vi "DSPS_E36000.Get ID.vi"(8 "error in":errorcluster, 11 "VISA Alias":refnum<visa-resource-name>) -> (0 "error out":errorcluster, 1 "SN":string, 2 "Model":string, 3 "VISA Alias Dup":refnum<visa-resource-name>, 4 "FW":string, 5 "Mfg":string)   [LabVIEW 2018]
panel:
  out "IDN Data":string
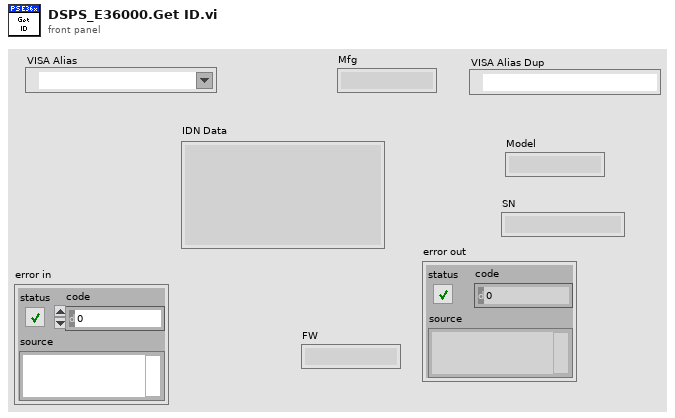
[diagram p1: front panel]
types:
  T1 = cluster{"Mfg":string, "Model":string, "SN":string, "FW":string}
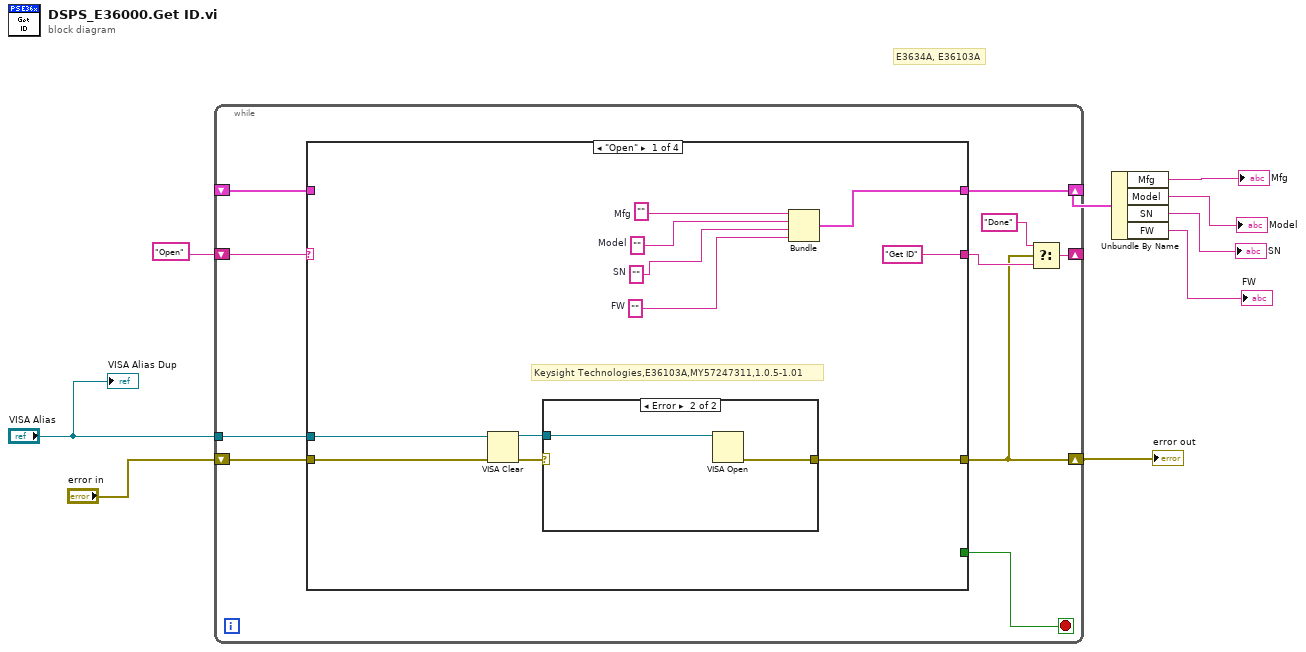
[diagram p0: block diagram]
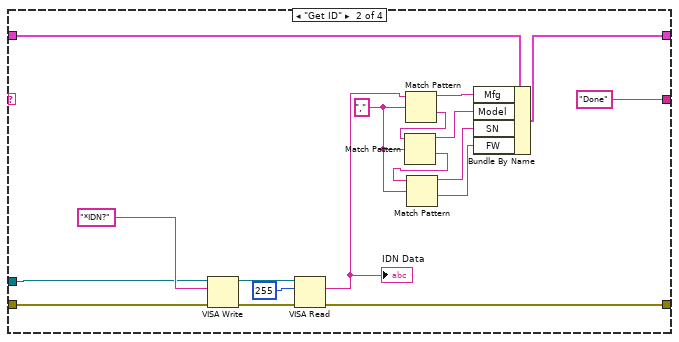
[diagram p3: hidden frame]
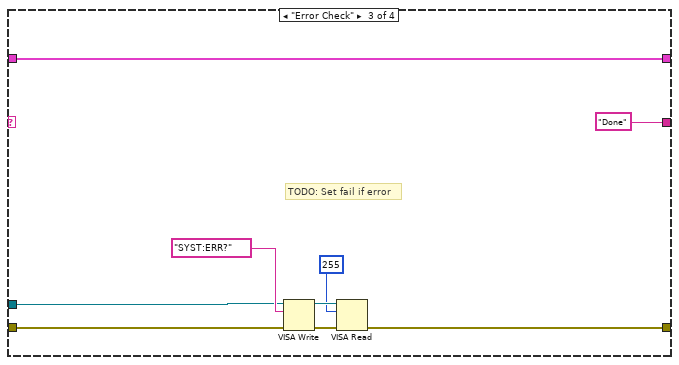
[diagram p4: hidden frame]
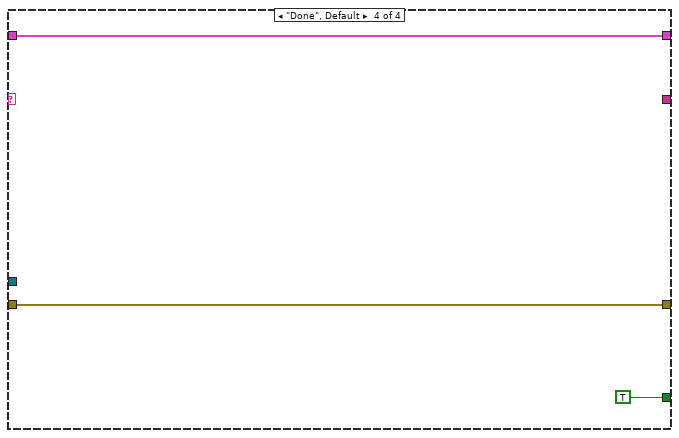
[diagram p5: hidden frame]
diagram:
  # "E3634A, E36103A"
  n1 = while {
    shift-right: [w15] -> w5
    shift-left: _ -> [w18]
    shift-right: [w12] -> _
    shift-left: "Open" -> [w19]
    tunnel: "VISA Alias" -> [w17]
    shift-right: [w11] -> w6
    shift-left: "error in" -> [w16]
    stop <- w10 stop-if-true
    n2 = case shown="\"Open\"" w19 {
      tunnel: w18 -> [_ w47 w53 w62]
      tunnel: w17 -> [w24 w50 w56 _]
      tunnel: w16 -> [w23 w49 w54 w61]
      tunnel: [w20 w43 w55 w61] -> w11
      tunnel: [w30 w46 w53 w62] -> w15
      tunnel: ["Get ID" "Done" "Done" _] -> w13
      tunnel: [_ _ _ TRUE] -> w10
      frame "Open" {
        w25 = ""  # FW
        w26 = ""  # SN
        w27 = ""  # Model
        w28 = ""  # Mfg
        # "Keysight Technologies,E36103A,MY57247311,1.0.5-1.01"
        n3 = VISA Clear(VISA resource name=w24, error in (no error)=w23) -> (VISA resource name out=w21:refnum<visa-resource-name>, error out=w22:errorcluster)
        n4 = case shown="Error" w22 {
          selector: w22 -> [w31 _]
          tunnel: w21 -> [_ w32]
          tunnel: [w31 w33] -> w20
          frame No Error {
          }
          frame Error {
            n5 = VISA Open(VISA resource name=w32) -> (error out=w33:errorcluster)  [unwired: 4 in, 1 out]
          }
        }
        n6 = Bundle("Mfg"=w28, "Model"=w27, "SN"=w26, "FW"=w25) -> (w30:T1)  [unwired: 1 in]
      }
      frame "Get ID" {
        w37 = ","
        n7 = VISA Write(VISA resource name=w50, write buffer="*IDN?", error in (no error)=w49) -> (VISA resource name out=w45:refnum<visa-resource-name>, error out=w44:errorcluster)  [unwired: 1 out]
        n8 = VISA Read(VISA resource name=w45, byte count=u32 255, error in (no error)=w44) -> (read buffer=w38:string, error out=w43:errorcluster)  [unwired: 2 out]
        "IDN Data" <- w38
        n9 = Match Pattern(string=w38, regular expression=w37) -> (before substring=w41:string, after substring=w40:string)  [unwired: 1 in, 2 out]
        n10 = Match Pattern(string=w40, regular expression=w37) -> (before substring=w39:string, after substring=w36:string)  [unwired: 1 in, 2 out]
        n11 = Match Pattern(string=w36, regular expression=w37) -> (before substring=w35:string, after substring=w34:string)  [unwired: 1 in, 2 out]
        n12 = Bundle By Name(cluster=w47, "Mfg"=w41, "Model"=w39, "SN"=w35, "FW"=w34) -> (w46:T1)
      }
      frame "Error Check" {
        # "TODO: Set fail if error"
        n13 = VISA Write(VISA resource name=w56, write buffer="SYST:ERR?", error in (no error)=w54) -> (VISA resource name out=w60:refnum<visa-resource-name>, error out=w58:errorcluster)  [unwired: 1 out]
        n14 = VISA Read(VISA resource name=w60, byte count=u32 255 ("byte count (0)"), error in (no error)=w58) -> (error out=w55:errorcluster)  [unwired: 3 out]
      }
      frame "Done", Default {
      }
    }
    n15 = Select(t="Done", s=w11, f=w13) -> (s? t:f=w12:string)
  }
  "error out" <- w6
  n16 = Unbundle By Name(w5) -> ("Mfg"=→"Mfg":string, "Model"=→"Model":string, "SN"=→"SN":string, "FW"=→"FW":string)
  "VISA Alias Dup" <- "VISA Alias"
